vi "Pressure Conversion.vi"(8 "error in (no error)":errorcluster, 10 "Voltage":dbl, 11 "APG in":refnum<class "APG.lvclass">) -> (0 "error out":errorcluster, 2 "Pressure":dbl)   [LabVIEW 2021, in "APG.lvclass"]
uses:
  APG.lvclass
  APG.lvclass/APG.ctl
  5fc59121-b0ef-4822-8bb0-24664bec5372.vi
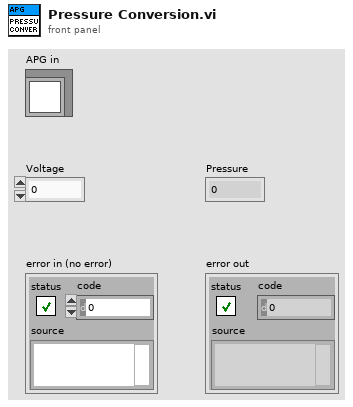
[diagram p1: front panel]
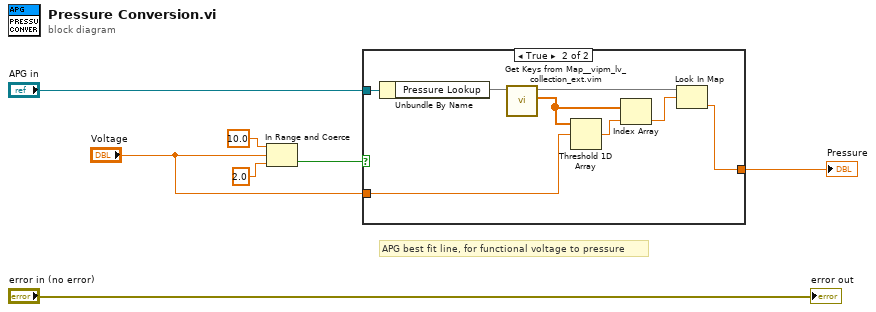
[diagram p0: block diagram]
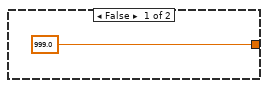
[diagram p2: hidden frame]
diagram:
  # "APG best fit line, for functional voltage to pressure"
  n1 = In Range and Coerce(upper limit=10.0, x="Voltage", lower limit=2.0) -> (In Range?=w3:bool)  [unwired: 1 out]
  n2 = case shown="True" w3 {
    tunnel: "APG in" -> [_ w16]
    tunnel: [999.0 ("Pressure") w15] -> w6
    tunnel: "Voltage" -> [_ w13]
    frame False {
    }
    frame True {
      n3 = Unbundle By Name(w16) -> ("Pressure Lookup"=w9:map{dbl, dbl})
      n4 = call "Get Keys from Map__vipm_lv_collection_ext.vim"("map"=w9) -> ("keys"=w12:dbl[], "map out"=w14:map{dbl, dbl})  [unwired: 9 in]
      n5 = Threshold 1D Array(2:w13, 3:w12) -> (0:w11:dbl)  [unwired: 1 in]
      n6 = Index Array(array=w12, index=w11) -> (element=w10:dbl)
      n7 = Look In Map(map=w14, key=w10) -> (value=w15:dbl)  [unwired: 1 in, 1 out]
    }
  }
  "Pressure" <- w6
  "error out" <- "error in (no error)"
